vi "log analysis_gps.vi"() -> ()   [LabVIEW 2018] (continued)
0 0\trobot status\t173.474266\t120.437413\t7.932300\t-1.472038\t-1.222257\t-0.266116\t0.000000\t0.000000\n\t\n15:16:16.7\tlog_raw\tgps_raw\t\tsystem status\tnormal 2 28.200000 0 0\trobot status\t173.473948\t120.438150\t7.930300\t-1.471516\t-1.220709\t-0.267182\t0.000000\t0.000000\n\t\n15:16:17.2\tlog_raw\tgps_raw\t\tsystem status\tnormal 2 28.200000 0 0\trobot status\t173.473795\t120.438831\t7.928600\t-1.468291\t-1.221393\t-0.269271\t0.000000\t0.000000\n\t\n15:16:17.7\tlog_raw\tgps_raw\t\tsystem status\tnormal 2 28.200000 0 0\trobot status\t173.473515\t120.439683\t7.926800\t-1.465481\t-1.220701\t-0.269691\t0.000000\t0.000000\n\t\n15:16:18.2\tlog_raw\tgps_raw\t#INSPVAXA,USB3,0,48.0,FINESTEERING,2107,281796.200,02000000,471d,15824;INS_ALIGNMENT_COMPLETE,INS_RTKFIXED,37.37121541125,126.72279352515,7.9254,22.3000,-0.0002,0.0035,0.0060,-1.463145311,-1.218768654,90.268956721,0.2548,0.1854,0.3737,0.0345,0.0343,0.0314,0.1516,0.1493,5.0350,0f000005,0*63f626df\n\tsystem status\tnormal 2 28.200000 0 0\trobot status\t173.473641\t120.440327\t7.925400\t-1.463145\t-1.218769\t-0.268957\t0.000000\t0.000000\n\t\n15:16:18.7\tlog_raw\tgps_raw\t\tsystem status\tnormal 2 28.200000 0 0\trobot status\t173.473988\t120.440220\t7.924400\t-1.461725\t-1.219842\t-0.268340\t0.000000\t0.000000\n\t\n15:16:19.2\tlog_raw\tgps_raw\t\tsystem status\tnormal 2 28.100000 0 0\trobot status\t173.482554\t120.439777\t7.924200\t-1.436035\t-1.015885\t-0.101255\t0.234000\t-0.043000\n\t\n15:16:19.7\tlog_raw\tgps_raw\t#INSPVAXA,USB3,0,43.0,FINESTEERING,2107,281797.700,02000000,471d,15824;INS_ALIGNMENT_COMPLETE,INS_RTKFIXED,37.37121541556,126.72279591257,7.9222,22.3000,-0.0052,0.3417,0.0085,-1.766936692,-1.171645490,90.396175106,0.2469,0.1802,0.3627,0.0345,0.0343,0.0313,0.1515,0.1492,5.0303,0f000005,0*2970234a\n\tsystem status\tnormal 2 28.200000 0 0\trobot status\t173.685115\t120.440801\t7.922200\t-1.766937\t-1.171645\t-0.396175\t0.317000\t0.082000\n\t\n15:16:20.2\tlog_raw\tgps_raw\t\tsystem status\tnormal 2 28.200000 0 0\trobot status\t173.799568\t120.438648\t7.922000\t-1.752408\t-1.164786\t-0.540243\t0.299000\t-0.021000\n\t\n15:16:20.7\tlog_raw\tgps_raw\t#INSPVAXA,USB3,0,45.5,FINESTEERING,2107,281798.700,02000000,471d,15824;INS_ALIGNMENT_COMPLETE,INS_RTKFIXED,37.37121535057,126.72279879079,7.9235,22.3000,-0.0085,0.3000,0.0138,-1.696631834,-1.054944377,90.699133923,0.2423,0.1802,0.3574,0.0527,0.0471,0.0400,0.1536,0.1513,5.0319,0f000001,0*b28cf3b5\n\tsystem status\tnormal 2 28.200000 0 0\trobot status\t173.940063\t120.433583\t7.923500\t-1.696632\t-1.054944\t-0.699134\t0.302000\t-0.014000\n\t\n15:16:21.2\tlog_raw\tgps_raw\t\tsystem status\tnormal 2 28.200000 0 0\trobot status\t174.076665\t120.428136\t7.925500\t-1.593958\t-0.917146\t-0.828214\t0.296000\t-0.019000\n\t\n15:16:21.7\tlog_raw\tgps_raw\t\tsystem status\tnormal 2 28.200000 0 0\trobot status\t174.225756\t120.422917\t7.928700\t-1.749923\t-0.980209\t-1.083801\t0.305000\t-0.014000\n\t\n15:16:22.2\tlog_raw\tgps_raw\t#INSPVAXA,USB3,0,46.0,FINESTEERING,2107,281800.200,02000000,471d,15824;INS_ALIGNMENT_COMPLETE,INS_RTKFIXED,37.37121518346,126.72280384244,7.9320,22.3000,-0.0138,0.3041,-0.0020,-1.831014383,-0.921017115,91.358421751,0.2498,0.2023,0.3609,0.0772,0.0698,0.0531,0.1576,0.1555,5.0235,0f000001,0*fd249ab4\n\tsystem status\tnormal 2 28.200000 0 0\trobot status\t174.387529\t120.415027\t7.932000\t-1.831014\t-0.921017\t-1.358422\t0.298000\t-0.021000\n\t\n15:16:22.7\tlog_raw\tgps_raw\t\tsystem status\tnormal 2 28.200000 0 0\trobot status\t174.520234\t120.407016\t7.934500\t-1.880751\t-0.785508\t-1.600367\t0.281000\t-0.031000\n\t\n15:16:23.2\tlog_raw\tgps_raw\t\tsystem status\tnormal 2 28.100000 0 0\trobot status\t174.667002\t120.396244\t7.937300\t-1.899959\t-0.808216\t-2.072579\t0.288000\t-0.024000\n\t\n15:16:23.7\tlog_raw\tgps_raw\t#INSPVAXA,USB3,0,45.0,FINESTEERING,2107,281801.700,02008000,471d,15824;INS_ALIGNMENT_COMPLETE,INS_RTKFIXED,37.37121487597,126.72280876147,7.9415,22.3000,-0.0281,0.2809,0.0050,-1.870107911,-0.684128774,92.617548886,0.2701,0.2229,0.3702,0.0875,0.0787,0.0583,0.1591,0.1573,5.0044,0f000001,0*b89165ad\n\tsystem status\tnormal 2 28.100000 0 0\trobot status\t174.823249\t120.380891\t7.941500\t-1.870108\t-0.684129\t-2.617549\t0.358000\t0.079000\n\t\n15:16:24.2\tlog_raw\tgps_raw\t\tsystem status\tnormal 2 28.100000 0 0\trobot status\t174.951604\t120.366363\t7.946000\t-1.872405\t-0.506334\t-3.242495\t0.380000\t0.102000\n\t\n15:16:24.7\tlog_raw\tgps_raw\t#INSPVAXA,USB3,0,48.0,FINESTEERING,2107,281802.700,02008000,471d,15824;INS_ALIGNMENT_COMPLETE,INS_RTKFIXED,37.37121453908,126.72281198538,7.9511,22.3000,-0.0315,0.2792,0.0111,-1.788436181,-0.484915836,93.932977011,0.2978,0.2449,0.3840,0.0951,0.0852,0.0628,0.1602,0.1589,4.9745,0f000001,0*1b429bef\n\tsystem status\tnormal 2 28.100000 0 0\trobot status\t175.108818\t120.343495\t7.951100\t-1.788436\t-0.484916\t-3.932977\t0.246000\t-0.086000\n\t\n15:16:25.2\tlog_raw\tgps_raw\t\tsystem status\tnormal 2 28.100000 0 0\trobot status\t175.237172\t120.322273\t7.955600\t-1.683644\t-0.414048\t-4.497819\t0.308000\t-0.011000\n\t\n15:16:25.7\tlog_raw\tgps_raw\t\tsystem status\tnormal 2 28.100000 0 0\trobot status\t175.376828\t120.295392\t7.960100\t-1.575532\t-0.418409\t-5.044426\t0.370000\t0.089000\n\t\n15:16:26.2\tlog_raw\tgps_raw\t#INSPVAXA,USB3,0,48.5,FINESTEERING,2107,281804.200,02008000,471d,15824;INS_ALIGNMENT_COMPLETE,INS_RTKFIXED,37.37121383035,126.72281674518,7.9651,22.3000,-0.0315,0.2774,0.0174,-1.651879586,-0.284385340,95.400888665,0.3536,0.2781,0.4212,0.1050,0.0912,0.0696,0.1611,0.1606,4.9104,0f000001,0*27f05722\n\tsystem status\tnormal 2 28.200000 0 0\trobot status\t175.530433\t120.264828\t7.965100\t-1.651880\t-0.284385\t-5.400889\t0.278000\t-0.039000\n\t\n15:16:26.7\tlog_raw\tgps_raw\t#INSPVAXA,USB3,0,48.5,FINESTEERING,2107,281804.700,02008000,471d,15824;INS_ALIGNMENT_COMPLETE,INS_RTKFIXED,37.37121355118,126.72281832287,7.9691,22.3000,-0.0490,0.2623,0.0114,-1.600367868,-0.284854057,95.675635132,0.3536,0.2781,0.4212,0.1050,0.0912,0.0696,0.1611,0.1606,4.9104,0f000001,0*fdce50cc\n\tsystem status\tnormal 2 28.200000 0 0\trobot status\t175.670182\t120.233842\t7.969100\t-1.600368\t-0.284854\t-5.675635\t0.283000\t-0.025000\n\t\n15:16:27.2\tlog_raw\tgps_raw\t\tsystem status\tnormal 2 28.200000 0 0\trobot status\t175.789678\t120.205150\t7.973700\t-1.464641\t-0.362171\t-5.857795\t0.303000\t0.000000\n\t\n15:16:27.7\tlog_raw\tgps_raw\t\tsystem status\tnormal 2 28.200000 0 0\trobot status\t175.923046\t120.174062\t7.979000\t-1.283152\t-0.301330\t-6.007293\t0.298000\t0.023000\n\t\n15:16:28.2\tlog_raw\tgps_raw\t#INSPVAXA,USB3,0,47.5,FINESTEERING,2107,281806.200,02000000,471d,15824;INS_ALIGNMENT_COMPLETE,INS_RTKFIXED,37.37121269576,126.72282281458,7.9853,22.3000,-0.0549,0.2699,0.0235,-1.099815041,-0.190468307,96.163961880,0.3893,0.2926,0.4618,0.1082,0.0921,0.0739,0.1610,0.1610,4.8764,0f000001,0*3796a6d3\n\tsystem status\tnormal 2 28.200000 0 0\trobot status\t176.068050\t120.138895\t7.985300\t-1.099815\t-0.190468\t-6.163962\t0.296000\t0.017000\n\t\n15:16:28.7\tlog_raw\tgps_raw\t\tsystem status\tnormal 2 28.200000 0 0\trobot status\t176.193699\t120.109860\t7.990400\t-1.018137\t-0.208161\t-6.197932\t0.296000\t0.023000\n\t\n15:16:29.2\tlog_raw\tgps_raw\t#INSPVAXA,USB3,0,49.0,FINESTEERING,2107,281807.200,02000000,471d,15824;INS_ALIGNMENT_COMPLETE,INS_RTKFIXED,37.37121211278,126.72282605036,7.9969,22.3000,-0.0568,0.3027,0.0138,-1.053067803,-0.177291074,96.270087858,0.3995,0.2955,0.4805,0.1085,0.0920,0.0753,0.1609,0.1610,4.8712,0f000001,0*6bce3c8a\n\tsystem status\tnormal 2 28.100000 0 0\trobot status\t176.354671\t120.074187\t7.996900\t-1.053068\t-0.177291\t-6.270088\t0.304000\t0.024000\n\t\n15:16:29.7\tlog_raw\tgps_raw\t#INSPVAXA,USB3,0,49.0,FINESTEERING,2107,281807.700,02000000,471d,15824;INS_ALIGNMENT_COMPLETE,INS_RTKFIXED,37.37121182995,126.72282768938,8.0018,22.3000,-0.0581,0.2574,0.0176,-1.058374656,-0.238658340,96.102791514,0.3995,0.2955,0.4805,0.1085,0.0920,0.0753,0.1609,0.1610,4.8712,0f000001,0*be10ea19\n\tsystem status\tnormal 2 28.100000 0 0\trobot status\t176.499852\t120.042794\t8.001800\t-1.058375\t-0.238658\t-6.102792\t0.329000\t-0.034000\n\t\n15:16:30.2\tlog_raw\tgps_raw\t#INSPVAXA,USB3,0,50.0,FINESTEERING,2107,281808.200,02000000,471d,15824;INS_ALIGNMENT_COMPLETE,INS_RTKFIXED,37.37121156109,126.72282925658,8.0066,22.3000,-0.0729,0.2643,0.0186,-0.872363263,-0.172820983,95.527165768,0.4058,0.2969,0.4970,0.1085,0.0920,0.0762,0.1608,0.1609,4.8702,0f000001,0*2e1aa4d5\n\tsystem status\tnormal 2 28.100000 0 0\trobot status\t176.638672\t120.012952\t8.006600\t-0.872363\t-0.172821\t-5.527166\t0.352000\t-0.050000\n\t\n15:16:30.7\tlog_raw\tgps_raw\t\tsystem status\tnormal 2 28.000000 0 0\trobot status\t176.762016\t119.988938\t8.010700\t-0.702147\t-0.254371\t-4.907782\t0.268000\t0.087000\n\t\n15:16:31.2\tlog_raw\tgps_raw\t\tsystem status\tnormal 2 27.900000 0 0\trobot status\t176.896014\t119.964557\t8.013800\t-0.597491\t-0.400071\t-3.772814\t0.221000\t0.162000\n\t\n15:16:31.7\tlog_raw\tgps_raw\t\tsystem status\tnormal 2 27.800000 0 0\trobot status\t177.035034\t119.943266\t8.015900\t-0.494749\t-0.530357\t-2.324093\t0.305000\t0.053000\n\t\n15:16:32.2\tlog_raw\tgps_raw\t\tsystem status\tnormal 2 27.800000 0 0\trobot status\t177.173780\t119.927361\t8.017800\t-0.643926\t-0.585190\t-1.121919\t0.303000\t0.040000\n\t\n15:16:32.7\tlog_raw\tgps_raw\t#INSPVAXA,USB3,0,47.5,FINESTEERING,2107,281810.700,02000000,471d,15824;INS_ALIGNMENT_COMPLETE,INS_RTKFIXED,37.37121067103,126.72283703860,8.0191,22.3000,-0.0356,0.2756,0.0276,-0.647693750,-0.582187036,89.865016518,0.4124,0.2979,0.5229,0.1081,0.0920,0.0770,0.1607,0.1609,4.8726,0f000001,0*855b65fe\n\tsystem status\tnormal 2 27.800000 0 0\trobot status\t177.327991\t119.914155\t8.019100\t-0.647694\t-0.582187\t0.134983\t0.309000\t0.029000\n\t\n15:16:33.2\tlog_raw\tgps_raw\t#INSPVAXA,USB3,0,45.5,FINESTEERING,2107,281811.200,02000000,471d,15824;INS_ALIGNMENT_COMPLETE,INS_RTKFIXED,37.37121058449,126.72283863071,8.0196,22.3000,-0.0335,0.2776,0.0134,-0.642436462,-0.620062849,88.791539404,0.4132,0.2980,0.5319,0.1079,0.0921,0.0771,0.1607,0.1609,4.8738,0f000001,0*5d2242c7\n\tsystem status\tnormal 2 27.900000 0 0\trobot status\t177.469017\t119.904547\t8.019600\t-0.642436\t-0.620063\t1.208461\t0.300000\t0.023000\n\t\n15:16:33.7\tlog_raw\tgps_raw\t#INSPVAXA,USB3,0,45.5,FINESTEERING,2107,281811.700,02000000,471d,15824;INS_ALIGNMENT_COMPLETE,INS_RTKFIXED,37.37121052303,126.72284024830,8.0190,22.3000,-0.0385,0.2808,0.0125,-0.613070377,-0.534497293,88.053265281,0.4132,0.2980,0.5319,0.1079,0.0921,0.0771,0.1607,0.1609,4.8738,0f000001,0*21e07958\n\tsystem status\tnormal 2 27.900000 0 0\trobot status\t177.612301\t119.897723\t8.019000\t-0.613070\t-0.534497\t1.946735\t0.302000\t0.032000\n\t\n15:16:34.2\tlog_raw\tgps_raw\t#INSPVAXA,USB3,0,48.5,FINESTEERING,2107,281812.200,02000000,471d,15824;INS_ALIGNMENT_COMPLETE,INS_RTKFIXED,37.37121047493,126.72284184822,8.0183,22.3000,-0.0314,0.2883,0.0148,-0.539418931,-0.410155130,87.563487932,0.4135,0.2980,0.5387,0.1083,0.0923,0.0770,0.1607,0.1609,4.8744,0f000001,0*aee609c3\n\tsystem status\tnormal 2 28.000000 0 0\trobot status\t177.754019\t119.892381\t8.018300\t-0.539419\t-0.410155\t2.436512\t0.341000\t-0.041000\n\t\n15:16:34.7\tlog_raw\tgps_raw\t#INSPVAXA,USB3,0,48.5,FINESTEERING,2107,281812.700,02000000,471d,15824;INS_ALIGNMENT_COMPLETE,INS_RTKFIXED,37.37121044769,126.72284347413,8.0176,22.3000,-0.0247,0.2718,0.0203,-0.569551057,-0.519035178,87.323829382,0.4135,0.2980,0.5387,0.1083,0.0923,0.0770,0.1607,0.1609,4.8744,0f000001,0*0b29fab3\n\tsystem status\tnormal 2 28.000000 0 0\trobot status\t177.898040\t119.889355\t8.017600\t-0.569551\t-0.519035\t2.676171\t0.434000\t-0.201000\n\t\n15:16:35.2\tlog_raw\tgps_raw\t#INSPVAXA,USB3,0,49.5,FINESTEERING,2107,281813.200,02000000,471d,15824;INS_ALIGNMENT_COMPLETE,INS_RTKFIXED,37.37121043009,126.72284509802,8.0163,22.3000,-0.0270,0.2716,0.0250,-0.708149800,-0.786508619,87.284677212,0.4137,0.2982,0.5437,0.1082,0.0926,0.0769,0.1607,0.1609,4.8743,0f000001,0*3e525f31\n\tsystem status\tnormal 2 28.100000 0 0\trobot status\t178.041881\t119.887399\t8.016300\t-0.708150\t-0.786509\t2.715323\t0.249000\t0.069000\n\t\n15:16:35.7\tlog_raw\tgps_raw\t#INSPVAXA,USB3,0,49.5,FINESTEERING,2107,281813.700,02000000,471d,15824;INS_ALIGNMENT_COMPLETE,INS_RTKFIXED,37.37121041419,126.72284671710,8.0139,22.3000,-0.0269,0.2730,0.0206,-0.734434421,-0.847262919,87.384621044,0.4137,0.2982,0.5437,0.1082,0.0926,0.0769,0.1607,0.1609,4.8743,0f000001,0*ad1d52fd\n\tsystem status\tnormal 2 28.100000 0 0\trobot status\t178.185297\t119.885631\t8.013900\t-0.734434\t-0.847263\t2.615379\t0.247000\t0.063000\n\t\n15:16:36.2\tlog_raw\tgps_raw\t#INSPVAXA,USB3,0,51.5,FINESTEERING,2107,281814.200,02000000,471d,15824;INS_ALIGNMENT_COMPLETE,INS_RTKFIXED,37.37121039679,126.72284831835,8.0121,22.3000,-0.0282,0.2780,0.0157,-0.723695017,-0.718771223,87.478292195,0.4133,0.2982,0.5471,0.1087,0.0929,0.0768,0.1607,0.1609,4.8744,0f000001,0*2471b93a\n\tsystem status\tnormal 2 28.200000 0 0\trobot status\t178.327133\t119.883697\t8.012100\t-0.723695\t-0.718771\t2.521708\t0.299000\t-0.016000\n\t\n15:16:36.7\tlog_raw\tgps_raw\t#INSPVAXA,USB3,0,51.5,FINESTEERING,2107,281814.700,02000000,471d,15824;INS_ALIGNMENT_COMPLETE,INS_RTKFIXED,37.37121037596,126.72284994702,8.0093,22.3000,-0.0392,0.2745,0.0084,-0.653618450,-0.794919707,87.628354192,0.4133,0.2982,0.5471,0.1087,0.0929,0.0768,0.1607,0.1609,4.8744,0f000001,0*e403a187\n\tsystem status\tnormal 2 28.200000 0 0\trobot status\t178.471398\t119.881382\t8.009300\t-0.653618\t-0.794920\t2.371646\t0.298000\t-0.025000\n\t\n15:16:37.2\tlog_raw\tgps_raw\t#INSPVAXA,USB3,0,48.5,FINESTEERING,2107,281815.200,02000000,471d,15824;INS_ALIGNMENT_COMPLETE,INS_RTKFIXED,37.37121035462,126.72285153134,8.0061,22.3000,-0.0298,0.2645,0.0056,-0.689462144,-0.765571273,87.819585359,0.4135,0.2983,0.5496,0.1092,0.0931,0.0767,0.1607,0.1609,4.8745,0f000001,0*3d6e9c36\n\tsystem status\tnormal 2 28.200000 0 0\trobot status\t178.611734\t119.879011\t8.006100\t-0.689462\t-0.765571\t2.180415\t0.296000\t-0.026000\n\t\n15:16:37.7\tlog_raw\tgps_raw\t#INSPVAXA,USB3,0,48.5,FINESTEERING,2107,281815.700,02000000,471d,15824;INS_ALIGNMENT_COMPLETE,INS_RTKFIXED,37.37121033500,126.72285311005,8.0032,22.3000,-0.0264,0.2987,0.0158,-0.781716650,-0.583090906,88.033249941,0.4135,0.2983,0.5496,0.1092,0.0931,0.0767,0.1607,0.1609,4.8745,0f000001,0*4dfcf1d6\n\tsystem status\tnormal 2 28.100000 0 0\trobot status\t178.751574\t119.876830\t8.003200\t-0.781717\t-0.583091\t1.966750\t0.296000\t-0.033000\n\t\n15:16:38.2\tlog_raw\tgps_raw\t#INSPVAXA,USB3,0,51.0,FINESTEERING,2107,281816.200,02008000,471d,15824;INS_ALIGNMENT_COMPLETE,INS_RTKFIXED,37.37121030517,126.72285487145,8.0002,22.3000,-0.0425,0.2860,0.0120,-0.722434536,-0.707507472,88.283028579,0.4136,0.2984,0.5510,0.1094,0.0933,0.0766,0.1607,0.1609,4.8747,0f000001,0*7939fe65\n\tsystem status\tnormal 2 28.200000 0 0\trobot status\t178.907596\t119.873516\t8.000200\t-0.722435\t-0.707507\t1.716971\t0.299000\t-0.018000\n\t\n15:16:38.7\tlog_raw\tgps_raw\t#INSPVAXA,USB3,0,51.0,FINESTEERING,2107,281816.700,02008000,471d,15824;INS_ALIGNMENT_COMPLETE,INS_RTKFIXED,37.37121027801,126.72285655609,7.9980,22.3000,-0.0398,0.3098,0.0245,-0.754705884,-0.828367575,88.621683950,0.4136,0.2984,0.5510,0.1094,0.0933,0.0766,0.1607,0.1609,4.8747,0f000001,0*590aa229\n\tsystem status\tnormal 2 28.100000 0 0\trobot status\t179.056818\t119.870498\t7.998000\t-0.754706\t-0.828368\t1.378316\t0.309000\t-0.025000\n\t\n15:16:39.2\tlog_raw\tgps_raw\t#INSPVAXA,USB3,0,48.5,FINESTEERING,2107,281817.200,02008000,471d,15824;INS_ALIGNMENT_COMPLETE,INS_RTKFIXED,37.37121021919,126.72285821539,7.9935,22.3000,-0.0399,0.3049,0.0009,-0.558805216,-0.866819508,89.180337786,0.4133,0.2986,0.5518,0.1098,0.0934,0.0766,0.1606,0.1608,4.8755,0f000001,0*c032cfc0\n\tsystem status\tnormal 2 28.100000 0 0\trobot status\t179.203796\t119.863967\t7.993500\t-0.558805\t-0.866820\t0.819662\t0.380000\t0.080000\n\t\n15:16:39.7\tlog_raw\tgps_raw\t#INSPVAXA,USB3,0,48.5,FINESTEERING,2107,281817.700,02008000,471d,15824;INS_ALIGNMENT_COMPLETE,INS_RTKFIXED,37.37121014797,126.72285990079,7.9875,22.3000,-0.0366,0.2866,-0.0014,-0.542824992,-1.209169915,90.078081458,0.4133,0.2986,0.5518,0.1098,0.0934,0.0766,0.1606,0.1608,4.8755,0f000001,0*9b0194b0\n\tsystem status\tnormal 2 28.100000 0 0\trobot status\t179.353086\t119.856060\t7.987500\t-0.542825\t-1.209170\t-0.078081\t0.297000\t-0.038000\n\t\n15:16:40.2\tlog_raw\tgps_raw\t#INSPVAXA,USB3,0,48.0,FINESTEERING,2107,281818.200,02008000,471d,15824;INS_ALIGNMENT_COMPLETE,INS_RTKFIXED,37.37121006905,126.72286154850,7.9830,22.3000,-0.0357,0.2838,0.0134,-0.818598247,-1.286018630,91.179102857,0.4133,0.2987,0.5521,0.1099,0.0933,0.0766,0.1606,0.1607,4.8765,0f000001,0*fb948376\n\tsystem status\tnormal 2 27.900000 0 0\trobot status\t179.499038\t119.847298\t7.983000\t-0.818598\t-1.286019\t-1.179103\t0.246000\t-0.118000\n\t\n15:16:40.7\tlog_raw\tgps_raw\t#INSPVAXA,USB3,0,48.0,FINESTEERING,2107,281818.700,02008000,471d,15824;INS_ALIGNMENT_COMPLETE,INS_RTKFIXED,37.37120996329,126.72286319027,7.9792,22.3000,-0.0377,0.2984,0.0070,-0.940731055,-1.250722578,92.396481410,0.4133,0.2987,0.5521,0.1099,0.0933,0.0766,0.1606,0.1607,4.8765,0f000001,0*0f67b83c\n\tsystem status\tnormal 2 27.900000 0 0\trobot status\t179.644463\t119.835557\t7.979200\t-0.940731\t-1.250723\t-2.396481\t0.292000\t-0.060000\n\t\n15:16:41.2\tlog_raw\tgps_raw\t#INSPVAXA,USB3,0,49.0,FINESTEERING,2107,281819.200,02008000,471d,15824;INS_ALIGNMENT_COMPLETE,INS_RTKFIXED,37.37120981052,126.72286484515,7.9750,22.3000,-0.0478,0.2879,0.0099,-0.798984239,-1.444181950,93.568970081,0.4129,0.2987,0.5522,0.1099,0.0932,0.0766,0.1605,0.1605,4.8778,0f000001,0*6b031fe9\n\tsystem status\tnormal 2 27.900000 0 0\trobot status\t179.791050\t119.818599\t7.975000\t-0.798984\t-1.444182\t-3.568970\t0.226000\t-0.140000\n\t\n15:16:41.7\tlog_raw\tgps_raw\t#INSPVAXA,USB3,0,49.0,FINESTEERING,2107,281819.700,02008000,471d,15824;INS_ALIGNMENT_COMPLETE,INS_RTKFIXED,37.37120962300,126.72286650676,7.9705,22.3000,-0.0671,0.2946,0.0135,-0.649128294,-1.472904568,94.664078192,0.4129,0.2987,0.5522,0.1099,0.0932,0.0766,0.1605,0.1605,4.8778,0f000001,0*2bf58c7b\n\tsystem status\tnormal 2 27.900000 0 0\trobot status\t179.938232\t119.797784\t7.970500\t-0.649128\t-1.472905\t-4.664078\t0.282000\t-0.046000\n\t\n15:16:42.2\tlog_raw\tgps_raw\t#INSPVAXA,USB3,0,48.5,FINESTEERING,2107,281820.200,02008000,471d,15824;INS_ALIGNMENT_COMPLETE,INS_RTKFIXED,37.37120940139,126.72286814747,7.9651,22.3000,-0.0641,0.2873,0.0149,-0.504838875,-1.441095327,95.746291084,0.4127,0.2987,0.5521,0.1098,0.0930,0.0766,0.1605,0.1604,4.8792,0f000001,0*7c1d55f3\n\tsystem status\tnormal 2 28.000000 0 0\trobot status\t180.083564\t119.773185\t7.965100\t-0.504839\t-1.441095\t-5.746291\t0.321000\t0.009000\n\t\n15:16:42.7\tlog_raw\tgps_raw\t#INSPVAXA,USB3,0,48.5,FINESTEERING,2107,281820.700,02008000,471d,15824;INS_ALIGNMENT_COMPLETE,INS_RTKFIXED,37.37120917103,126.72286978921,7.9589,22.3000,-0.0688,0.2879,0.0058,-0.603273984,-1.593663516,96.633630255,0.4127,0.2987,0.5521,0.1098,0.0930,0.0766,0.1605,0.1604,4.8792,0f000001,0*e21ec5f9\n\tsystem status\tnormal 2 28.000000 0 0\trobot status\t180.228986\t119.747616\t7.958900\t-0.603274\t-1.593664\t-6.633630\t0.286000\t-0.039000\n\t\n15:16:43.2\tlog_raw\tgps_raw\t#DUALANTENNAHEADINGA,USB3,0,48.5,FINESTEERING,2107,281821.200,02000000,d426,15824;SOL_COMPUTED,NARROW_FLOAT,-1.000000000,199.802429199,59.611751556,0.0,103.871536255,169.545913696,\"631T\",19,8,8,8,04,00,20,23*e0db817a\n\tsystem status\tnormal 2 28.100000 0 0\trobot status\t180.374669\t119.720702\t7.953700\t-0.715360\t-1.645902\t-7.242907\t0.331000\t0.033000\n\t\n15:16:43.7\tlog_raw\tgps_raw\t#INSPVAXA,USB3,0,48.5,FINESTEERING,2107,281821.700,02000000,471d,15824;INS_ALIGNMENT_COMPLETE,INS_RTKFIXED,37.37120867107,126.72287305353,7.9486,22.3000,-0.0854,0.2737,-0.0020,-0.718036711,-1.580500229,97.593601208,0.4126,0.2986,0.5520,0.1098,0.0929,0.0766,0.1604,0.1603,4.8804,0f000001,0*a82ce81c\n\tsystem status\tnormal 2 28.100000 0 0\trobot status\t180.518134\t119.692121\t7.948600\t-0.718037\t-1.580500\t-7.593601\t0.292000\t-0.011000\n\t\n15:16:44.2\tlog_raw\tgps_raw\t#INSPVAXA,USB3,0,51.0,FINESTEERING,2107,281822.200,02000000,471d,15824;INS_ALIGNMENT_COMPLETE,INS_RTKFIXED,37.37120839710,126.72287464148,7.9433,22.3000,-0.0737,0.2706,0.0058,-0.493099711,-1.491040971,97.883869188,0.4123,0.2985,0.5518,0.1098,0.0930,0.0767,0.1604,0.1602,4.8814,0f000001,0*43cf4a7f\n\tsystem status\tnormal 2 28.200000 0 0\trobot status\t180.658792\t119.661712\t7.943300\t-0.493100\t-1.491041\t-7.883869\t0.412000\t0.173000\n\t\n15:16:44.7\tlog_raw\tgps_raw\t#DUALANTENNAHEADINGA,USB3,0,51.0,FINESTEERING,2107,281822.700,02000000,d426,15824;SOL_COMPUTED,NARROW_FLOAT,-1.000000000,199.656448364,63.340484619,0.0,99.066596985,82.183616638,\"631T\",18,8,8,8,04,00,20,23*3eb0b03b\n\tsystem status\tnormal 2 28.200000 0 0\trobot status\t180.799616\t119.631740\t7.938700\t-0.479394\t-1.326314\t-8.025813\t0.289000\t-0.007000\n\t\n15:16:45.2\tlog_raw\tgps_raw\t#INSPVAXA,USB3,0,46.0,FINESTEERING,2107,281823.200,02000000,471d,15824;INS_ALIGNMENT_COMPLETE,INS_RTKFIXED,37.37120785592,126.72287776108,7.9348,22.3000,-0.0813,0.2968,0.0005,-0.426101177,-1.082566624,98.131503900,0.4122,0.2985,0.5517,0.1098,0.0931,0.0768,0.1603,0.1602,4.8821,0f000001,0*e97d0866\n\tsystem status\tnormal 2 28.200000 0 0\trobot status\t180.935121\t119.601643\t7.934800\t-0.426101\t-1.082567\t-8.131504\t0.299000\t0.013000\n\t\n15:16:45.7\tlog_raw\tgps_raw\t#DUALANTENNAHEADINGA,USB3,0,46.0,FINESTEERING,2107,281823.700,02000000,d426,15824;SOL_COMPUTED,NARROW_FLOAT,-1.000000000,152.081710815,66.315963745,0.0,360.000000000,174.707107544,\"631T\",18,9,9,8,04,00,20,23*2d86097d\n\tsystem status\tnormal 2 28.200000 0 0\trobot status\t181.082130\t119.569420\t7.931500\t-0.316038\t-1.151321\t-8.250547\t0.301000\t0.017000\n\t\n15:16:46.2\tlog_raw\tgps_raw\t#DUALANTENNAHEADINGA,USB3,0,50.0,FINESTEERING,2107,281824.200,02000000,d426,15824;SOL_COMPUTED,NARROW_FLOAT,-1.000000000,155.447463989,72.039955139,0.0,360.000000000,145.525100708,\"631T\",18,9,9,8,04,00,20,23*f6d7a9cd\n\tsystem status\tnormal 2 28.200000 0 0\trobot status\t181.221261\t119.538481\t7.928800\t-0.297661\t-1.153969\t-8.324516\t0.301000\t0.016000\n\t\n15:16:46.7\tlog_raw\tgps_raw\t#INSPVAXA,USB3,0,50.0,FINESTEERING,2107,281824.700,02000000,471d,15824;INS_ALIGNMENT_COMPLETE,INS_RTKFIXED,37.37120702523,126.72288248256,7.9286,22.3000,-0.1000,0.2970,-0.0030,-0.414363931,-1.319109492,98.317764432,0.4124,0.2984,0.5515,0.1099,0.0933,0.0768,0.1603,0.1602,4.8829,0f000001,0*6aa4622c\n\tsystem status\tnormal 2 28.200000 0 0\trobot status\t181.353342\t119.509440\t7.928600\t-0.414364\t-1.319109\t-8.317764\t0.297000\t0.015000\n\t\n15:16:47.2\tlog_raw\tgps_raw\t#DUALANTENNAHEADINGA,USB3,0,49.5,FINESTEERING,2107,281825.200,02000000,d426,15824;SOL_COMPUTED,L1_FLOAT,-1.000000000,69.256408691,12.160554886,0.0,285.962799072,180.000000000,\"631T\",19,8,8,5,04,00,20,21*0683b703\n\tsystem status\tnormal 2 28.100000 0 0\trobot status\t181.493500\t119.478559\t7.930600\t-0.498119\t-0.963634\t-8.321892\t0.286000\t0.019000\n\t\n15:16:47.7\tlog_raw\tgps_raw\t#INSPVAXA,USB3,0,49.5,FINESTEERING,2107,281825.700,02000000,471d,15824;INS_ALIGNMENT_COMPLETE,INS_RTKFIXED,37.37120646463,126.72288578375,7.9281,22.3000,-0.0763,0.2904,0.0216,-0.793323324,-0.889298592,98.320200190,0.4125,0.2985,0.5514,0.1101,0.0934,0.0769,0.1602,0.1602,4.8839,0f000001,0*5f866581\n\tsystem status\tnormal 2 28.100000 0 0\trobot status\t181.645756\t119.447216\t7.928100\t-0.793323\t-0.889299\t-8.320200\t0.347000\t-0.058000\n\t\n15:16:48.2\tlog_raw\tgps_raw\t#INSPVAXA,USB3,0,48.5,FINESTEERING,2107,281826.200,02000000,471d,15824;INS_ALIGNMENT_COMPLETE,INS_RTKFIXED,37.37120619057,126.72288730405,7.9253,22.3000,-0.0749,0.2848,0.0194,-0.697963338,-0.472482314,97.902378657,0.4129,0.2985,0.5514,0.1102,0.0935,0.0770,0.1601,0.1601,4.8852,0f000001,0*4b4d602c\n\tsystem status\tnormal 2 28.100000 0 0\trobot status\t181.780422\t119.416797\t7.925300\t-0.697963\t-0.472482\t-7.902379\t0.262000\t0.086000\n\t\n15:16:48.7\tlog_raw\tgps_raw\t#INSPVAXA,USB3,0,48.5,FINESTEERING,2107,281826.700,02000000,471d,15824;INS_ALIGNMENT_COMPLETE,INS_RTKFIXED,37.37120593844,126.72288885558,7.9222,22.3000,-0.0660,0.2989,0.0157,-0.925431746,0.038687863,97.361199599,0.4129,0.2985,0.5514,0.1102,0.0935,0.0770,0.1601,0.1601,4.8852,0f000001,0*d022d5ea\n\tsystem status\tnormal 2 28.000000 0 0\trobot status\t181.917854\t119.388811\t7.922200\t-0.925432\t0.038688\t-7.361200\t0.377000\t-0.090000\n\t\n15:16:49.2\tlog_raw\tgps_raw\t#DUALANTENNAHEADINGA,USB3,0,49.5,FINESTEERING,2107,281827.200,02000000,d426,15824;SOL_COMPUTED,NARROW_FLOAT,-1.000000000,106.272483826,69.863449097,0.0,360.000000000,180.000000000,\"631T\",18,5,5,5,04,00,20,03*ec53100b\n\tsystem status\tnormal 2 28.000000 0 0\trobot status\t182.053608\t119.364134\t7.919900\t-1.175042\t0.457085\t-6.511478\t0.254000\t0.080000\n\t\n15:16:49.7\tlog_raw\tgps_raw\t#INSPVAXA,USB3,0,49.5,FINESTEERING,2107,281827.700,02000000,471d,15824;INS_ALIGNMENT_COMPLETE,INS_RTKFIXED,37.37120552459,126.72289199783,7.9230,22.3000,-0.0613,0.2731,0.0106,-1.441869650,0.390097771,95.831538133,0.4135,0.2986,0.5515,0.1109,0.0937,0.0770,0.1599,0.1601,4.8868,0f000001,0*586a71ed\n\tsystem status\tnormal 2 28.000000 0 0\trobot status\t182.196189\t119.342874\t7.923000\t-1.441870\t0.390098\t-5.831538\t0.268000\t0.071000\n\t\n15:16:50.2\tlog_raw\tgps_raw\t#INSPVAXA,USB3,0,51.0,FINESTEERING,2107,281828.200,02000000,471d,15824;INS_ALIGNMENT_COMPLETE,INS_RTKFIXED,37.37120533257,126.72289355096,7.9234,22.3000,-0.0675,0.2814,0.0290,-1.476207155,0.673066178,94.890255810,0.4144,0.2985,0.5514,0.1108,0.0941,0.0770,0.1598,0.1600,4.8875,0f000001,0*65bdbb94\n\tsystem status\tnormal 2 27.800000 0 0\trobot status\t182.333763\t119.321560\t7.923400\t-1.476207\t0.673066\t-4.890256\t0.219000\t0.143000\n\t\n15:16:50.7\tlog_raw\tgps_raw\t#INSPVAXA,USB3,0,51.0,FINESTEERING,2107,281828.700,02000000,471d,15824;INS_ALIGNMENT_COMPLETE,INS_RTKFIXED,37.37120515804,126.72289518020,7.9256,22.3000,-0.0694,0.2933,0.0211,-1.265355938,0.544212560,94.152212733,0.4144,0.2985,0.5514,0.1108,0.0941,0.0770,0.1598,0.1600,4.8875,0f000001,0*3fa45f89\n\tsystem status\tnormal 2 27.900000 0 0\trobot status\t182.478079\t119.302187\t7.925600\t-1.265356\t0.544213\t-4.152213\t0.296000\t0.014000\n\t\n15:16:51.2\tlog_raw\tgps_raw\t#INSPVAXA,USB3,0,46.5,FINESTEERING,2107,281829.200,02000000,471d,15824;INS_ALIGNMENT_COMPLETE,INS_RTKFIXED,37.37120502580,126.72289678148,7.9278,22.3000,-0.0502,0.2768,0.0145,-1.429978780,0.528599128,93.605134571,0.4154,0.2985,0.5516,0.1105,0.0939,0.0771,0.1597,0.1599,4.8857,0f000001,0*990165b1\n\tsystem status\tnormal 2 27.900000 0 0\trobot status\t182.619917\t119.287507\t7.927800\t-1.429979\t0.528599\t-3.605135\t0.245000\t0.087000\n\t\n15:16:51.7\tlog_raw\tgps_raw\t#DUALANTENNAHEADINGA,USB3,0,46.5,FINESTEERING,2107,281829.700,02000000,d426,15824;SOL_COMPUTED,NARROW_FLOAT,-1.000000000,57.886253357,2.555429220,0.0,154.963073730,180.000000000,\"631T\",19,7,7,5,04,00,20,03*f9e0cff3\n\tsystem status\tnormal 2 27.900000 0 0\trobot status\t182.759519\t119.275374\t7.929800\t-1.665027\t0.569309\t-3.139732\t0.335000\t-0.036000\n\t\n15:16:52.2\tlog_raw\tgps_raw\t#DUALANTENNAHEADINGA,USB3,0,49.5,FINESTEERING,2107,281830.200,02000000,d426,15824;SOL_COMPUTED,L1_FLOAT,-1.000000000,83.986137390,10.132819176,0.0,360.000000000,180.000000000,\"631T\",19,6,6,3,04,00,20,01*1abfa712\n\tsystem status\tnormal 2 28.000000 0 0\trobot status\t182.901440\t119.260719\t7.932500\t-1.450747\t0.438012\t-2.716418\t0.397000\t-0.149000\n\t\n15:16:52.7\tlog_raw\tgps_raw\t#INSPVAXA,USB3,0,49.5,FINESTEERING,2107,281830.700,02000000,471d,15824;INS_ALIGNMENT_COMPLETE,INS_RTKFIXED,37.37120465229,126.72290157166,7.9350,22.3000,-0.0442,0.2947,0.0242,-1.334244960,0.390910805,92.567102853,0.4155,0.2984,0.5517,0.1101,0.0937,0.0771,0.1595,0.1599,4.8819,0f000001,0*e118fdc5\n\tsystem status\tnormal 2 28.100000 0 0\trobot status\t183.044224\t119.246044\t7.935000\t-1.334245\t0.390911\t-2.567103\t0.281000\t0.040000\n\t\n15:16:53.2\tlog_raw\tgps_raw\t#DUALANTENNAHEADINGA,USB3,0,50.0,FINESTEERING,2107,281831.200,02000000,d426,15824;SOL_COMPUTED,NARROW_FLOAT,-1.000000000,59.043685913,-28.864562988,0.0,170.366668701,180.000000000,\"631T\",18,8,8,7,04,00,20,23*14dad2b0\n\tsystem status\tnormal 2 28.100000 0 0\trobot status\t183.184415\t119.232878\t7.938600\t-1.402397\t0.385830\t-2.597915\t0.326000\t-0.048000\n\t\n15:16:53.7\tlog_raw\tgps_raw\t#DUALANTENNAHEADINGA,USB3,0,50.0,FINESTEERING,2107,281831.700,02000000,d426,15824;SOL_COMPUTED,NARROW_FLOAT,-1.000000000,59.094017029,-28.251525879,0.0,171.144256592,180.000000000,\"631T\",17,8,8,7,04,00,20,23*b1c96c44\n\tsystem status\tnormal 2 28.100000 0 0\trobot status\t183.329739\t119.219725\t7.941800\t-1.493011\t0.204732\t-2.686910\t0.277000\t0.004000\n\t\n15:16:54.2\tlog_raw\tgps_raw\t#DUALANTENNAHEADINGA,USB3,0,51.0,FINESTEERING,2107,281832.200,02000000,d426,15824;SOL_COMPUTED,NARROW_FLOAT,-1.000000000,147.351470947,72.022521973,0.0,360.000000000,180.000000000,\"631T\",17,7,7,7,04,00,20,23*e605d7f3\n\tsystem status\tnormal 2 28.100000 0 0\trobot status\t183.470332\t119.207465\t7.944800\t-1.579295\t0.162622\t-2.785029\t0.306000\t-0.011000\n\t\n15:16:54.7\tlog_raw\tgps_raw\t#DUALANTENNAHEADINGA,USB3,0,51.0,FINESTEERING,2107,281832.700,02000000,d426,15824;SOL_COMPUTED,NARROW_FLOAT,-1.000000000,140.025573730,68.472808838,0.0,360.000000000,180.000000000,\"631T\",16,7,7,7,04,00,20,23*882fbccd\n\tsystem status\tnormal 2 28.100000 0 0\trobot status\t183.600004\t119.196416\t7.948100\t-1.578073\t0.294436\t-2.834380\t0.296000\t-0.023000\n\t\n15:16:55.2\tlog_raw\tgps_raw\t#DUALANTENNAHEADINGA,USB3,0,50.5,FINESTEERING,2107,281833.200,02000000,d426,15824;SOL_COMPUTED,NARROW_FLOAT,-1.000000000,68.082496643,-11.763427734,0.0,169.499374390,180.000000000,\"631T\",18,9,9,7,04,00,20,23*031ca633\n\tsystem status\tnormal 2 28.200000 0 0\trobot status\t183.738365\t119.185544\t7.951300\t-1.630962\t0.289844\t-2.998611\t0.295000\t-0.029000\n\t\n15:16:55.7\tlog_raw\tgps_raw\t#DUALANTENNAHEADINGA,USB3,0,50.5,FINESTEERING,2107,281833.700,02000000,d426,15824;SOL_COMPUTED,NARROW_FLOAT,-1.000000000,67.931724548,-11.679229736,0.0,169.789916992,180.000000000,\"631T\",18,9,9,7,04,00,20,23*9183d900\n\tsystem status\tnormal 2 28.100000 0 0\trobot status\t183.884359\t119.172473\t7.954300\t-1.528447\t0.233972\t-3.226689\t0.304000\t-0.035000\n\t\n15:16:56.2\tlog_raw\tgps_raw\t#DUALANTENNAHEADINGA,USB3,0,47.0,FINESTEERING,2107,281834.200,02000000,d426,15824;SOL_COMPUTED,NARROW_FLOAT,-1.000000000,117.470924377,63.855136871,0.0,360.000000000,180.000000000,\"631T\",18,5,5,5,04,00,20,03*04244261\n\tsystem status\tnormal 2 28.100000 0 0\trobot status\t184.033170\t119.159506\t7.957400\t-1.530203\t0.341657\t-3.499959\t0.310000\t-0.021000\n\t\n15:16:56.7\tlog_raw\tgps_raw\t#INSPVAXA,USB3,0,47.0,FINESTEERING,2107,281834.700,02000000,471d,15824;INS_ALIGNMENT_COMPLETE,INS_RTKFIXED,37.37120376020,126.72291436834,7.9622,22.3000,-0.0339,0.2802,0.0380,-1.719157085,0.362405119,93.876835430,0.4140,0.2983,0.5521,0.1098,0.0930,0.0772,0.1595,0.1599,4.8699,0f000001,0*4c3c706d\n\tsystem status\tnormal 2 28.100000 0 0\trobot status\t184.177733\t119.147011\t7.962200\t-1.719157\t0.362405\t-3.876835\t0.277000\t-0.064000\n\t\n15:16:57.2\tlog_raw\tgps_raw\t#DUALANTENNAHEADINGA,USB3,0,49.5,FINESTEERING,2107,281835.200,02000000,d426,15824;SOL_COMPUTED,NARROW_FLOAT,-1.000000000,56.406482697,-13.603881836,0.0,133.707977295,180.000000000,\"631T\",17,6,6,5,04,00,20,03*0c459025\n\tsystem status\tnormal 2 28.100000 0 0\trobot status\t184.322804\t119.132996\t7.966200\t-1.785820\t0.234004\t-4.496784\t0.287000\t-0.048000\n\t\n15:16:57.7\tlog_raw\tgps_raw\t#DUALANTENNAHEADINGA,USB3,0,49.5,FINESTEERING,2107,281835.700,02000000,d426,15824;SOL_COMPUTED,NARROW_FLOAT,-1.000000000,56.377288818,-12.403900146,0.0,134.026809692,180.000000000,\"631T\",18,6,6,5,04,00,20,03*a9390bed\n\tsystem status\tnormal 2 28.000000 0 0\trobot status\t184.466445\t119.116277\t7.968200\t-1.809311\t0.080084\t-5.298649\t0.253000\t-0.090000\n\t\n15:16:58.2\tlog_raw\tgps_raw\t#INSPVAXA,USB3,0,49.5,FINESTEERING,2107,281836.200,02000000,471d,15824;INS_ALIGNMENT_COMPLETE,INS_RTKFIXED,37.37120330531,126.72291919762,7.9715,22.3000,-0.0485,0.2910,0.0305,-1.607227145,0.177759790,96.248616069,0.4130,0.2982,0.5522,0.1099,0.0930,0.0773,0.1596,0.1599,4.8709,0f000001,0*7239ccf3\n\tsystem status\tnormal 2 28.000000 0 0\trobot status\t184.605502\t119.096515\t7.971500\t-1.607227\t0.177760\t-6.248616\t0.264000\t-0.089000\n\t\n15:16:58.7\tlog_raw\tgps_raw\t#DUALANTENNAHEADINGA,USB3,0,49.5,FINESTEERING,2107,281836.700,02000000,d426,15824;SOL_COMPUTED,L1_FLOAT,-1.000000000,75.942611694,16.211278915,0.0,339.522399902,180.000000000,\"631T\",19,6,6,3,04,00,20,01*51b3f26e\n\tsystem status\tnormal 2 27.900000 0 0\trobot status\t184.744038\t119.075756\t7.975000\t-1.385086\t0.202626\t-7.312290\t0.354000\t0.039000\n\t\n15:16:59.2\tlog_raw\tgps_raw\t#DUALANTENNAHEADINGA,USB3,0,48.5,FINESTEERING,2107,281837.200,02000000,d426,15824;SOL_COMPUTED,L1_FLOAT,-1.000000000,80.771942139,6.980556488,0.0,360.000000000,180.000000000,\"631T\",20,5,5,2,04,00,20,01*7f238ca7\n\tsystem status\tnormal 2 27.900000 0 0\trobot status\t184.884823\t119.051321\t7.978300\t-1.308155\t0.085403\t-8.506121\t0.268000\t-0.113000\n\t\n15:16:59.7\tlog_raw\tgps_raw\t#DUALANTENNAHEADINGA,USB3,0,48.5,FINESTEERING,2107,281837.700,02000000,d426,15824;SOL_COMPUTED,L1_FLOAT,-1.000000000,81.947074890,7.586090088,0.0,360.000000000,180.000000000,\"631T\",19,5,5,2,04,00,20,01*fab92539\n\tsystem status\tnormal 2 27.900000 0 0\trobot status\t185.020847\t119.024638\t7.980500\t-1.454643\t0.101503\t-9.672002\t0.308000\t-0.042000\n\t\n15:17:00.2\tlog_raw\tgps_raw\t#DUALANTENNAHEADINGA,USB3,0,50.5,FINESTEERING,2107,281838.200,02000000,d426,15824;SOL_COMPUTED,NARROW_FLOAT,-1.000000000,70.339691162,-8.337524414,0.0,360.000000000,180.000000000,\"631T\",19,5,5,5,04,00,20,03*774b3c80\n\tsystem status\tnormal 2 27.900000 0 0\trobot status\t185.156234\t118.995321\t7.984500\t-1.605735\t0.103358\t-10.547145\t0.378000\t0.086000\n\t\n15:17:00.7\tlog_raw\tgps_raw\t#DUALANTENNAHEADINGA,USB3,0,50.5,FINESTEERING,2107,281838.700,02000000,d426,15824;SOL_COMPUTED,NARROW_FLOAT,-1.000000000,76.530433655,10.538305283,0.0,360.000000000,180.000000000,\"631T\",20,5,5,5,04,00,20,03*8a1753aa\n\tsystem status\tnormal 2 28.000000 0 0\trobot status\t185.291246\t118.962578\t7.988600\t-1.642981\t0.128538\t-11.296184\t0.339000\t0.033000\n\t\n15:17:01.2\tlog_raw\tgps_raw\t#DUALANTENNAHEADINGA,USB3,0,48.5,FINESTEERING,2107,281839.200,02000000,d426,15824;SOL_COMPUTED,NARROW_FLOAT,-1.000000000,124.470252991,58.985340118,0.0,360.000000000,180.000000000,\"631T\",20,7,7,7,04,00,20,23*a245761b\n\tsystem status\tnormal 2 28.000000 0 0\trobot status\t185.425540\t118.928646\t7.992100\t-1.671118\t0.117849\t-11.882973\t0.287000\t-0.042000\n\t\n15:17:01.7\tlog_raw\tgps_raw\t#DUALANTENNAHEADINGA,USB3,0,48.5,FINESTEERING,2107,281839.700,02000000,d426,15824;SOL_COMPUTED,NARROW_FLOAT,-1.000000000,152.317840576,70.615020752,0.0,360.000000000,180.000000000,\"631T\",18,5,5,5,04,00,20,03*7061d411\n\tsystem status\tnormal 2 28.100000 0 0\trobot status\t185.557836\t118.893509\t7.993800\t-1.693041\t0.203476\t-12.397641\t0.242000\t-0.092000\n\t\n15:17:02.2\tlog_raw\tgps_raw\t#DUALANTENNAHEADINGA,USB3,0,48.0,FINESTEERING,2107,281840.200,02000000,d426,15824;SOL_COMPUTED,L1_FLOAT,-1.000000000,81.231452942,8.750979424,0.0,360.000000000,180.000000000,\"631T\",18,6,6,3,04,00,20,01*4b849010\n\tsystem status\tnormal 2 28.100000 0 0\trobot status\t185.690236\t118.857914\t7.995600\t-1.868066\t0.241539\t-12.759477\t0.263000\t-0.048000\n\t\n15:17:02.7\tlog_raw\tgps_raw\t#DUALANTENNAHEADINGA,USB3,0,48.0,FINESTEERING,2107,281840.700,02000000,d426,15824;SOL_COMPUTED,L1_FLOAT,-1.000000000,82.520584106,5.924606323,0.0,360.000000000,180.000000000,\"631T\",18,6,6,3,04,00,20,01*b6060555\n\tsystem status\tnormal 2 28.100000 0 0\trobot status\t185.823315\t118.819365\t7.997400\t-1.956523\t0.122514\t-13.087286\t0.304000\t0.002000\n\t\n15:17:03.2\tlog_raw\tgps_raw\t#DUALANTENNAHEADINGA,USB3,0,49.0,FINESTEERING,2107,281841.200,02000000,d426,15824;SOL_COMPUTED,L1_FLOAT,-1.000000000,85.243263245,10.185308456,0.0,360.000000000,180.000000000,\"631T\",19,6,6,3,04,00,20,01*39a33d99\n\tsystem status\tnormal 2 28.100000 0 0\trobot status\t185.949377\t118.781449\t7.998600\t-1.937422\t0.061193\t-13.312107\t0.301000\t0.006000\n\t\n15:17:03.7\tlog_raw\tgps_raw\t#DUALANTENNAHEADINGA,USB3,0,49.0,FINESTEERING,2107,281841.700,02000000,d426,15824;SOL_COMPUTED,L1_FLOAT,-1.000000000,84.280883789,10.021371841,0.0,360.000000000,180.000000000,\"631T\",20,6,6,3,04,00,20,01*b97d95c9\n\tsystem status\tnormal 2 28.200000 0 0\trobot status\t186.078047\t118.742341\t7.998500\t-1.953845\t-0.074934\t-13.436444\t0.296000\t0.019000\n\t\n15:17:04.2\tlog_raw\tgps_raw\t#DUALANTENNAHEADINGA,USB3,0,49.5,FINESTEERING,2107,281842.200,02000000,d426,15824;SOL_COMPUTED,NARROW_FLOAT,-1.000000000,70.006813049,-31.901763916,0.0,210.151992798,180.000000000,\"631T\",17,7,7,5,04,00,20,03*5ed3d42a\n\tsystem status\tnormal 2 28.100000 0 0\trobot status\t186.204769\t118.702702\t7.999500\t-1.937910\t-0.101005\t-13.538631\t0.306000\t0.015000\n\t\n15:17:04.7\tlog_raw\tgps_raw\t#DUALANTENNAHEADINGA,USB3,0,49.5,FINESTEERING,2107,281842.700,02000000,d426,15824;SOL_COMPUTED,NARROW_FLOAT,-1.000000000,69.602676392,-30.153381348,0.0,208.420791626,180.000000000,\"631T\",17,7,7,5,04,00,20,03*0e8eebe2\n\tsystem status\tnormal 2 28.100000 0 0\trobot status\t186.337850\t118.661069\t8.000900\t-2.006623\t-0.040208\t-13.577752\t0.296000\t0.023000\n\t\n15:17:05.2\tlog_raw\tgps_raw\t#DUALANTENNAHEADINGA,USB3,0,49.5,FINESTEERING,2107,281843.200,02000000,d426,15824;SOL_COMPUTED,NARROW_FLOAT,-1.000000000,134.588546753,49.958206177,0.0,360.000000000,180.000000000,\"631T\",17,5,5,5,04,00,20,03*524a8851\n\tsystem status\tnormal 2 28.100000 0 0\trobot status\t186.476395\t118.617130\t8.001700\t-1.910917\t0.017415\t-13.574771\t0.304000\t0.012000\n\t\n15:17:05.7\tlog_raw\tgps_raw\t#DUALANTENNAHEADINGA,USB3,0,49.5,FINESTEERING,2107,281843.700,02000000,d426,15824;SOL_COMPUTED,NARROW_FLOAT,-1.000000000,111.024063110,4.724229813,0.0,360.000000000,180.000000000,\"631T\",17,5,5,5,04,00,20,03*868053f4\n\tsystem status\tnormal 2 28.100000 0 0\trobot status\t186.611322\t118.573373\t8.002200\t-1.677627\t0.230813\t-13.474204\t0.298000\t0.035000\n\t\n15:17:06.2\tlog_raw\tgps_raw\t#DUALANTENNAHEADINGA,USB3,0,50.0,FINESTEERING,2107,281844.200,02000000,d426,15824;SOL_COMPUTED,L1_FLOAT,-1.000000000,91.707588196,-1.773010254,0.0,360.000000000,180.000000000,\"631T\",17,6,6,3,04,00,20,01*2b557997\n\tsystem status\tnormal 2 28.100000 0 0\trobot status\t186.746611\t118.531462\t8.001700\t-1.635272\t0.239307\t-13.252191\t0.303000\t0.020000\n\t\n15:17:06.7\tlog_raw\tgps_raw\t\tsystem status\tnormal 2 28.000000 0 0\trobot status\t186.883065\t118.491686\t8.000300\t-1.618760\t0.104824\t-12.818155\t0.252000\t0.087000\n\t\n15:17:07.2\tlog_raw\tgps_raw\t\tsystem status\tnormal 2 28.000000 0 0\trobot status\t187.017467\t118.454924\t7.998800\t-1.813978\t0.058520\t-12.163678\t0.378000\t-0.086000\n\t\n15:17:07.7\tlog_raw\tgps_raw\t#DUALANTENNAHEADINGA,USB3,0,50.0,FINESTEERING,2107,281845.700,02000000,d426,15824;SOL_COMPUTED,NARROW_FLOAT,-1.000000000,48.226726532,-51.942321777,0.0,56.526073456,74.567710876,\"631T\",21,6,6,5,04,00,20,03*278cdd49\n\tsystem status\tnormal 2 27.900000 0 0\trobot status\t187.151924\t118.418044\t7.998300\t-1.744728\t-0.080184\t-11.260531\t0.254000\t0.107000\n\t\n15:17:08.2\tlog_raw\tgps_raw\t#DUALANTENNAHEADINGA,USB3,0,50.0,FINESTEERING,2107,281846.200,02000000,d426,15824;SOL_COMPUTED,L1_FLOAT,-1.000000000,98.548431396,11.085563660,0.0,360.000000000,180.000000000,\"631T\",20,6,6,3,04,00,20,01*4cd03511\n\tsystem status\tnormal 2 27.900000 0 0\trobot status\t187.291420\t118.382820\t7.997500\t
